vi "Assert Not Equal Type_Variant.vi"(5 "Assert Only? (F)":bool, 6 "error code (1)":i32=1, 7 "Label":string, 8 "error in (no error)":errorcluster, 10 "Y":variant, 11 "X":variant) -> (0 "error out":errorcluster)   [LabVIEW 2009, in "Caraya.lvlib" / "Assert.lvclass"]
doc: "Generates an error if the input condition is not met.\n\nThis method compares the value of the inputs, irrespective of the type representation.\nAsserts TRUE if input values are equal.\nAsserts FALSE otherwise.\n\nex: Two integer inputs of equal value but of different type representation (U8 and I32) will assert TRUE."
uses:
  Assert.lvclass
  <vilib>/Utility/VariantDataType/VariantType.lvlib
panel:
  # "Copyright © 2015 JKI All rights reserved.\n\nAuthor: Tomi Maila <tomi.maila@jki.net>\n\nThis library is provided \"AS IS\" ,WITHOUT WARRANTIES OR\nCONDITIONS OF ANY KIND, either express or implied.\n\nJKI -- jki.net"
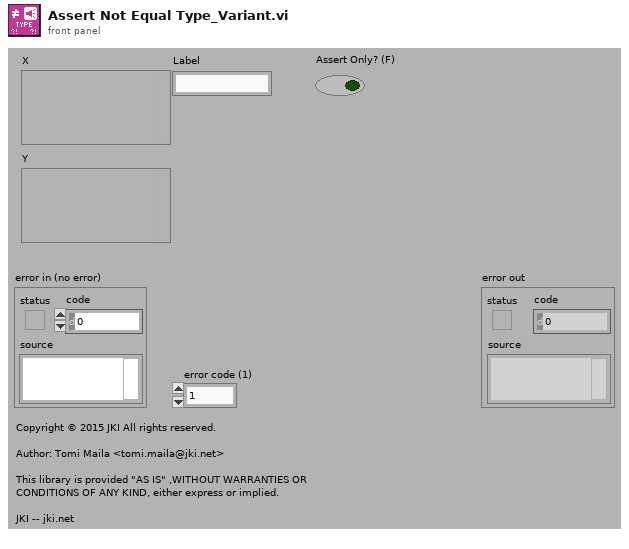
[diagram p1: front panel]
types:
  T1 = typedef "VariantType.lvlib/Type.ctl" = enum8{"Invalid Type", "Void", "I8", "I16", "I32", "I64", "U8", "U16", "U32", "U64", "Single Float", "Double Float", "Extended Float", "Single Complex", "Double Complex", "Extended Complex", "Enum U8", "Enum U16", "Enum U32", "Enum U64", "Single Float With Unit", "Double Float With Unit", "Extended Float With Unit", "Single Complex with Unit", "Double Complex with Unit", "Extended Complex with Unit", "Boolean", "String", "Path", "Picture", "Tag", "Array", "Cluster", "Variant", "LV Variant", "Waveform", "Timestamp", "Digital Waveform", "Digital Data", "ExpressData", "Refnum", "External Data", "VI", "Poly VI", "LabVIEW Class Instance", "Fixed Point"}
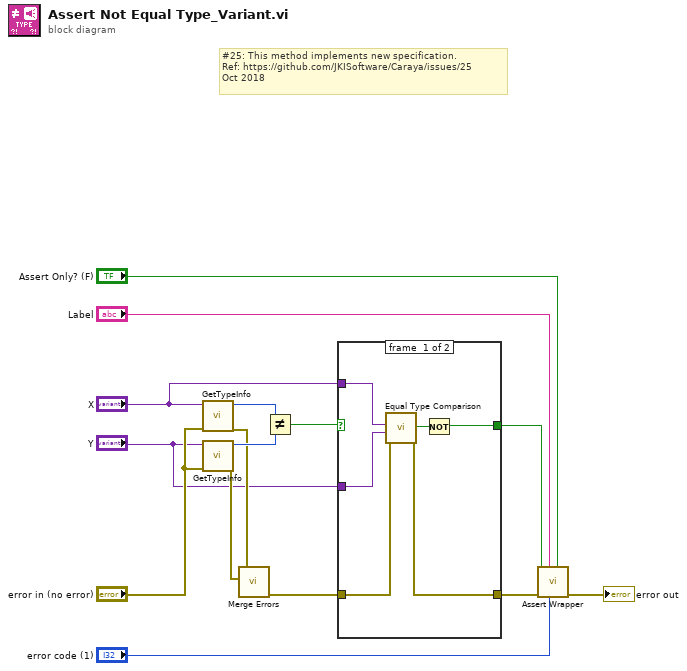
[diagram p0: block diagram]
diagram:
  # "#25: This method implements new specification.\nRef: https://github.com/JKISoftware/Caraya/issues/25\nOct 2018"
  n1 = call <vilib>:"GetTypeInfo.vi"("error in (no error)"="error in (no error)", "Variant"="X") -> ("error out"=w10:errorcluster, "Type Enum"=w8:T1)  [unwired: 5 in, 3 out]
  n2 = call <vilib>:"GetTypeInfo.vi"("error in (no error)"="error in (no error)", "Variant"="Y") -> ("error out"=w9:errorcluster, "Type Enum"=w11:T1)  [unwired: 5 in, 3 out]
  n3 = call <vilib>:"Merge Errors.vi"("error in 2 (no error)"=w9, "error in 1 (no error)"=w10) -> ("error out"=w3:errorcluster)  [unwired: 5 in]
  n4 = Not Equal?(x=w8, y=w11) -> (x != y?=w6:bool)
  n5 = case shown="False" w6 {
    selector: w6 -> [_ w23]
    tunnel: "X" -> [w21 _]
    tunnel: "Y" -> [w20 _]
    tunnel: w3 -> [w19 w22]
    tunnel: [w17 w23] -> w2
    tunnel: [w16 w22] -> w1
    frame #0 {
      n6 = call "Equal Type Comparison.vi"("error in (no error)"=w19, "Y"=w20, "X"=w21) -> ("error out"=w16:errorcluster, "Equal Types?"=w18:bool)  [unwired: 7 in]
      n7 = Not(x=w18) -> (.not. x?=w17:bool)
    }
    frame #1 {
    }
  }
  n8 = call "Assert Wrapper.vi"("Assert Only? (F)"="Assert Only? (F)", "error code (1)"="error code (1)", "Label"="Label", "error in (no error)"=w1, "Assert?"=w2) -> ("error out"=→"error out":errorcluster)  [unwired: 6 in]
